vi "Rasbperry Pi Compiler for LabVIEW Beta - Submit an Issue.vi"(8 "error in (no error)":errorcluster) -> (0 "error out":errorcluster)   [LabVIEW 2014, in "Raspberry Pi Compatible Compiler for LabVIEW.lvlib"]
uses:
  Raspberry Pi Compatible Compiler for LabVIEW.lvlib
  Custom Controls/Queue Message.ctl
panel:
  in  "User E-mail Address":string
  out "Animated Image":i16(ring) caption="Ring 2"
  in  "Exit":bool
  in  "Submit":bool
  in  "User Input":string caption="Description of the Issue and Steps to Reproduce"
  in  "Main VI Path":path caption="Path to the Top Level VI Causing the Issue"
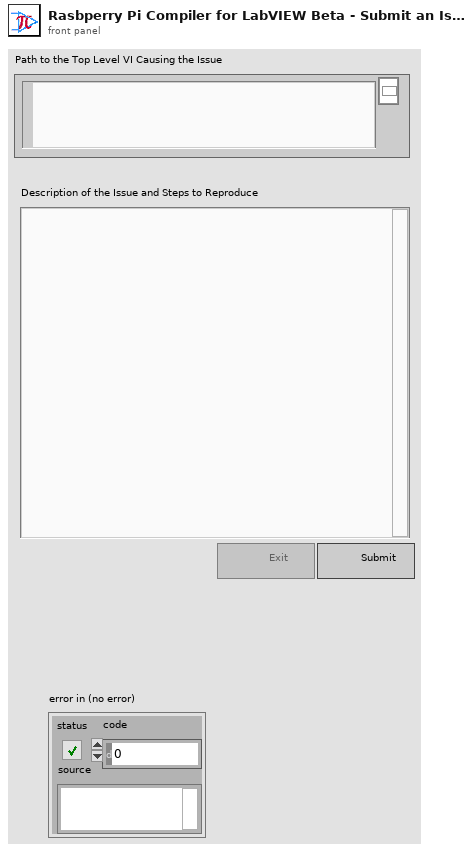
[diagram p1: front panel]
types:
  T1 = typedef "Raspberry Pi Compatible Compiler for LabVIEW.lvlib/Queue Message.ctl" = cluster{"Command":string, "Value":string}
  T2 = enum8{"Enabled", "Disabled", "Disabled and Grayed Out"}
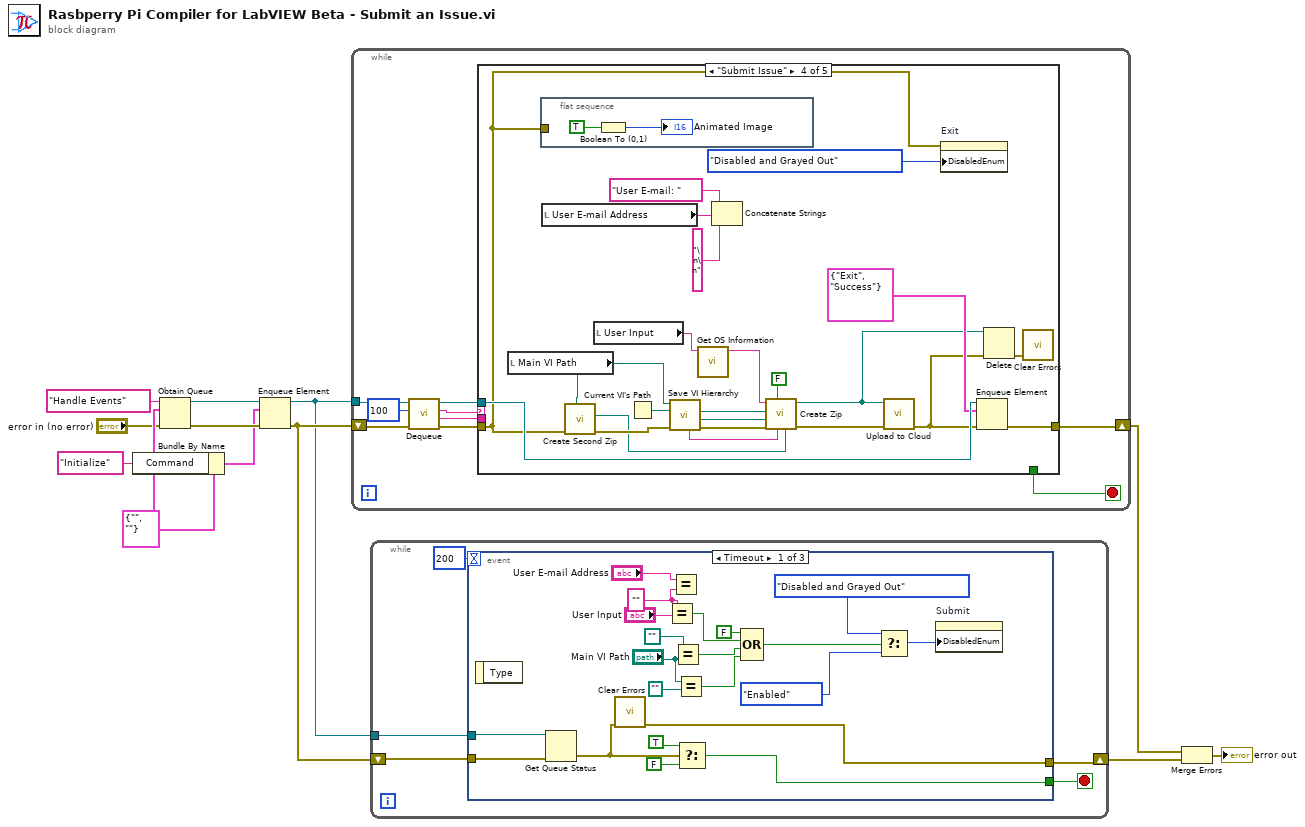
[diagram p0: block diagram]
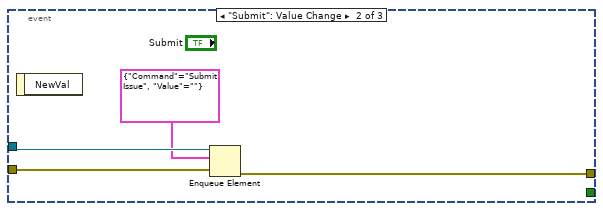
[diagram p2: hidden frame]
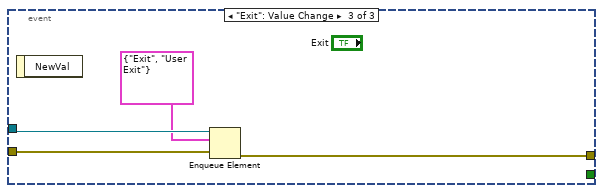
[diagram p3: hidden frame]
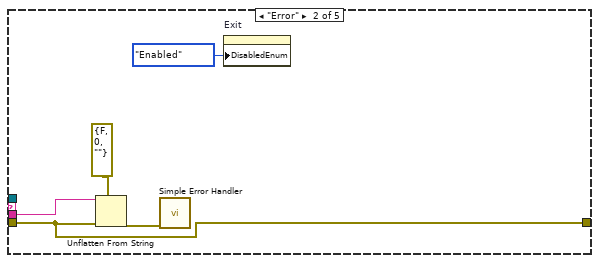
[diagram p5: hidden frame]
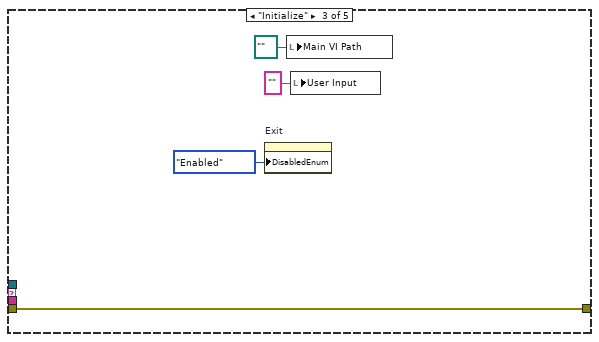
[diagram p6: hidden frame]
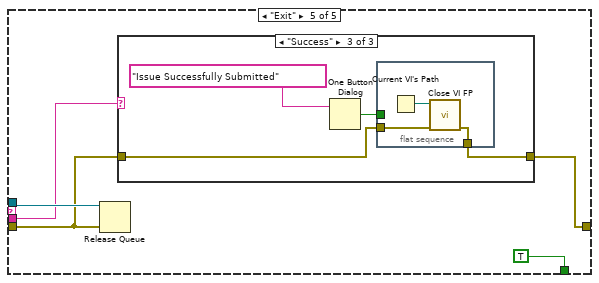
[diagram p7: hidden frame]
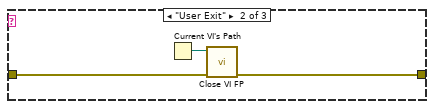
[diagram p9: hidden frame]
diagram:
  w9 = T1 {"Command"="", "Value"=""} ("Message")
  n1 = Bundle By Name(cluster=w9, "Command"="Initialize") -> (w8:T1)
  n2 = Obtain Queue(name (unnamed)="Handle Events", element data type=w9, error in (no error)="error in (no error)") -> (queue out=w10:refnum<queue>, error out=w11:errorcluster)  [unwired: 2 in, 1 out]
  n3 = Enqueue Element(queue=w10, element=w8, error in (no error)=w11) -> (queue out=w5:refnum<queue>, error out=w6:errorcluster)  [unwired: 1 in, 1 out]
  n4 = while {
    tunnel: w5 -> [w21]
    shift-right: [w13] -> w2
    shift-left: w6 -> [w20]
    stop <- w14 stop-if-true
    n5 = call "Dequeue.vi"("error in (no error)"=w20, "timeout in ms (100)"=100, "queue"=w21) -> ("error out"=w16:errorcluster, "Value"=w15:string, "Command"=w17:string, "queue out"=w18:refnum<queue>)  [unwired: 5 in]
    n6 = case shown="\"Submit Issue\"" w17 {
      tunnel: w18 -> [_ _ _ w47 w60]
      tunnel: w16 -> [w22 w26 w31 w35 w58]
      tunnel: w15 -> [_ w25 _ _ w59]
      tunnel: [_ _ _ _ TRUE] -> w14
      tunnel: [w22 w26 w31 w48 w57] -> w13
      frame "Idle", Default {
      }
      frame "Error" {
        n7 = Unflatten From String(type=errorcluster {"status"=FALSE, "code"=0, "source"=""} ("error in (no error)"), binary string=w25, error in (no error)=w26) -> (error out=w24:errorcluster)  [unwired: 4 out]
        n8 = call <vilib>:"Simple Error Handler.vi"("error in (no error)"=w24) -> ()  [unwired: 4 in, 5 out]
        n9 = property on="Exit" class="Bool"("DisabledEnum"=T2."Enabled" ("Disabled")) -> ()  [unwired: 2 in, 2 out]
      }
      frame "Initialize" {
        n10 = property on="Exit" class="Bool"("DisabledEnum"=T2."Enabled" ("Disabled")) -> ()  [unwired: 2 in, 2 out]
        n11 = local write "Main VI Path"(path "" ("Main VI Path")) -> ()
        n12 = local write "User Input"("" ("User Input")) -> ()
      }
      frame "Submit Issue" {
        n13 = local read "Main VI Path"() -> (w33:path)
        n14 = flat-sequence {
          tunnel: w35 -> [_]
          frame #0 {
            n15 = Boolean To (0,1)(Boolean=TRUE) -> (0, 1=→"Animated Image":i16)
          }
        }
        n16 = local read "User E-mail Address"() -> (w44:string)
        n17 = call "Create Second Zip.vi"("VIPath"=w33, "error in"=w35) -> ("error out"=w34:errorcluster, "Second ZIP"=w32:path)  [unwired: 8 in]
        n18 = local read "User Input"() -> (w40:string)
        n19 = Current VI's Path() -> (path=w54:path)
        n20 = call "Save VI Hierarchy.vi"("error in (no error)"=w34, "Current VI's Path"=w54, "Path to the Top Level VI Causing the Issue"=w33) -> ("error out"=w49:errorcluster, "Top Level Path"=w52:path, "Destination Directory"=w50:path, "Zip File Name"=w53:string)  [unwired: 5 in]
        n21 = call "Get OS Information.vi"("Steps to Reproduce"=w40) -> ("Metadata"=w39:string)  [unwired: 10 in]
        n22 = Concatenate Strings("User E-mail: " ("string"), w44, "\n\n" ("string")) -> ()  [unwired: 1 out]
        n23 = call "Create Zip.vi"("Second Zip"=w32, "ZIP File Name"=w53, "Generate MD5 File"=FALSE, "error in (no error)"=w49, "Top Level VI Path"=w52, "Destination Directory"=w50, "Metadata"=w39) -> ("error out"=w41:errorcluster, "Zip File Path"=w36:path)  [unwired: 3 in]
        n24 = call "Upload to Cloud.vi"("error in (no error)"=w41, "Zip File Path"=w36) -> ("error out"=w38:errorcluster)  [unwired: 9 in]
        n25 = property on="Exit" class="Bool"(error in=w35, "DisabledEnum"=T2."Disabled and Grayed Out" ("Disabled")) -> ()  [unwired: 1 in, 2 out]
        n26 = Enqueue Element(queue=w47, element=T1 {"Command"="Exit", "Value"="Success"}, error in (no error)=w38) -> (error out=w48:errorcluster)  [unwired: 1 in, 2 out]
        n27 = Delete(path (use dialog)=w36, error in=w38) -> (error out=w37:errorcluster)  [unwired: 3 in, 2 out]
        n28 = call <vilib>:"Clear Errors.vi"("error in (no error)"=w37) -> ()  [unwired: 5 in, 2 out]
      }
      frame "Exit" {
        n29 = Release Queue(queue=w60, error in (no error)=w58) -> ()  [unwired: 1 in, 3 out]
        n30 = case shown="\"Success\"" w59 {
          tunnel: w58 -> [w62 w64 w67]
          tunnel: [w62 w63 w66] -> w57
          frame "False", Default {
          }
          frame "User Exit" {
            n31 = Current VI's Path() -> (path=w65:path)
            n32 = call "Close VI FP.vi"("error in (no error)"=w64, "path"=w65) -> ("error out"=w63:errorcluster)  [unwired: 9 in]
          }
          frame "Success" {
            n33 = One Button Dialog(message="Issue Successfully Submitted") -> (true=w68:bool)  [unwired: 1 in]
            n34 = flat-sequence {
              tunnel: w68 -> [_]
              tunnel: w67 -> [w72]
              tunnel: [w71] -> w66
              frame #0 {
                n35 = Current VI's Path() -> (path=w70:path)
                n36 = call "Close VI FP.vi"("error in (no error)"=w72, "path"=w70) -> ("error out"=w71:errorcluster)  [unwired: 9 in]
              }
            }
          }
        }
      }
    }
  }
  n37 = while {
    tunnel: w5 -> [w77]
    shift-right: [w74] -> w3
    shift-left: w6 -> [w76]
    stop <- w75 stop-if-true
    n38 = event shown="[0] Timeout" {
      selector: _ -> [_ _ _]
      dyn-events: _ -> [_ _ _]
      timeout: 200 -> [_ _ _]
      tunnel: w77 -> [w98 w102 w106]
      tunnel: w76 -> [w97 w101 w105]
      tunnel: [w94 _ _] -> w75
      tunnel: [w92 w99 w103] -> w74
      event Timeout {
        w81 = "" ("x")
        n39 = event-data() -> ()  [unwired: 1 in, 1 out]
        n40 = Get Queue Status(queue=w98, error in (no error)=w97) -> (error out=w93:errorcluster)  [unwired: 1 in, 7 out]
        n41 = call <vilib>:"Clear Errors.vi"("error in (no error)"=w93) -> ("error out"=w92:errorcluster)  [unwired: 5 in, 1 out]
        n42 = Equal?(x=w81, y="User Input") -> (x = y?=w83:bool)
        n43 = Equal?(x="User E-mail Address", y=w81) -> ()  [unwired: 1 out]
        n44 = Equal?(x=path "", y="Main VI Path") -> (x = y?=w80:bool)
        n45 = Equal?(x="Main VI Path", y=path "") -> (x = y?=w79:bool)
        n46 = Select(t=TRUE, s=w93, f=FALSE) -> (s? t:f=w94:bool)
        n47 = Compound Arithmetic op=OR(FALSE ("value"), w83, w80, w79) -> (w87:bool)
        n48 = Select(t=T2."Disabled and Grayed Out", s=w87, f=T2."Enabled" ("Disabled")) -> (s? t:f=w85:T2)
        n49 = property on="Submit" class="Bool"("DisabledEnum"=w85) -> ()  [unwired: 2 in, 2 out]
      }
      event "Submit": Value Change {
        n50 = event-data() -> ()  [unwired: 1 in, 1 out]
        n51 = Enqueue Element(queue=w102, element=T1 {"Command"="Submit Issue", "Value"=""}, error in (no error)=w101) -> (error out=w99:errorcluster)  [unwired: 1 in, 2 out]
      }
      event "Exit": Value Change {
        n52 = event-data() -> ()  [unwired: 1 in, 1 out]
        n53 = Enqueue Element(queue=w106, element=T1 {"Command"="Exit", "Value"="User Exit"}, error in (no error)=w105) -> (error out=w103:errorcluster)  [unwired: 1 in, 2 out]
      }
    }
  }
  n54 = Merge Errors(w2, w3) -> (→"error out":errorcluster)
